vi "CTRE_PigeonIMU_Open.vi"   [LabVIEW 2016]
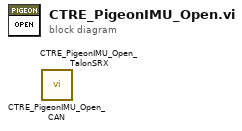
[diagram p0: block diagram]
diagram:
  n1 = call <vilib>:"CTRE_PigeonIMU_Open_CAN.vi"() -> ()  [unwired: 10 in, 2 out]
  n2 = call <vilib>:"CTRE_PigeonIMU_Open_TalonSRX.vi"() -> ()  [unwired: 10 in, 2 out]
